vi "Join Responses.vi"(1 "External Out":dbl[](array[numeric]), 2 "LBCB Number":T1, 3 "Response In":dbl[](array[numeric]), 4 "Servo\nError":dbl[](array[numeric]), 5 "Load\nCells":dbl[](array[numeric]), 6 "LVDTs":dbl[](array[numeric])) -> (0 "Responses Out":dbl[](array[numeric]))   [LabVIEW 2013]
uses:
  Data Access Objects/Metadata/LBCB Number.ctl
  Data Access Objects/Metadata/Persistant DAO Actions.ctl
  Data Access Objects/Application/Number Of LBCBs.ctl
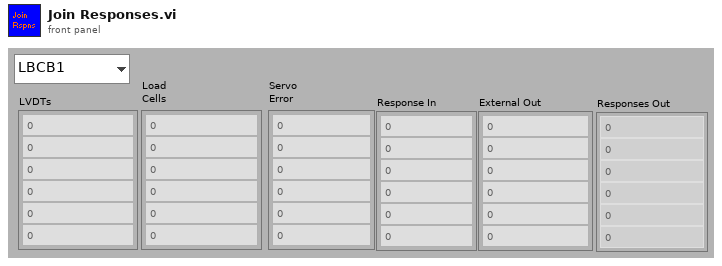
[diagram p1: front panel]
types:
  T1 = typedef "LBCB Number.ctl" = enum16{"LBCB1", "LBCB2"}
  T2 = typedef "Number Of LBCBs.ctl" = enum16{"1", "2"}
  T3 = typedef "Persistant DAO Actions.ctl" = enum16{"Init", "Get", "Set", "Load", "Save"}
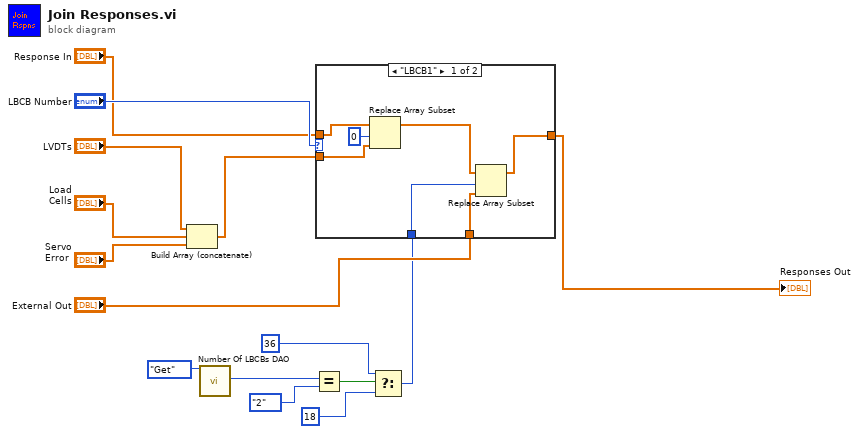
[diagram p0: block diagram]
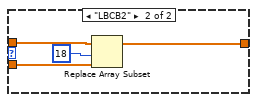
[diagram p2: hidden frame]
diagram:
  n1 = Build Array (concatenate)("LVDTs", "Load\nCells", "Servo\nError") -> (w11:dbl[])
  n2 = call "Number Of LBCBs DAO.vi"("Actions"=Persistant_DAO_Actions."Get") -> ("Number of\nLBCBs Out"=w6:T2)  [unwired: 13 in, 5 out]
  n3 = Equal?(x=w6, y=Number_Of_LBCBs."2") -> (x = y?=w4:bool)
  n4 = Select(t=36 ("index"), s=w4, f=18) -> (s? t:f=w2:i32)
  n5 = case shown="\"LBCB1\"" "LBCB Number" {
    tunnel: w11 -> [w20 w26]
    tunnel: "Response In" -> [w22 w25]
    tunnel: [w17 w23] -> w13
    tunnel: "External Out" -> [w19 _]
    tunnel: w2 -> [w16 _]
    frame "LBCB1" {
      n6 = Replace Array Subset(array=w22, new element=w20, index=0) -> (w18:dbl[])
      n7 = Replace Array Subset(array=w18, new element=w19, index=w16) -> (w17:dbl[])
    }
    frame "LBCB2" {
      n8 = Replace Array Subset(array=w25, new element=w26, index=18) -> (w23:dbl[])
    }
  }
  "Responses Out" <- w13
